vi "Read Motion Settings.vi"(8 "error in (no error)":errorcluster, 11 "Focus Class in":refnum<class "Focus Class.lvclass">) -> (0 "error out":errorcluster, 2 "Motion Settings":T1, 3 "Focus Class out":refnum<class "Focus Class.lvclass">)   [LabVIEW 2021, in "Focus Class.lvclass"]
uses:
  Focus Class.lvclass
  Focus cluster Motion Settings.ctl
  Focus Class.lvclass/Focus Class.ctl
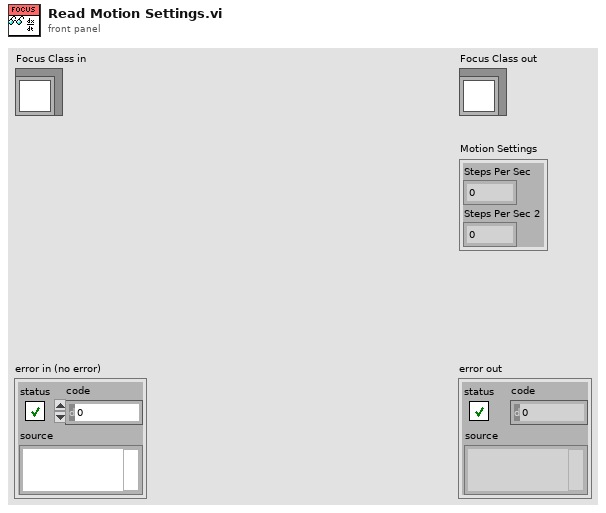
[diagram p1: front panel]
types:
  T1 = typedef "Focus cluster Motion Settings.ctl" = cluster{"Steps Per Sec":i32, "Steps Per Sec 2":i32}
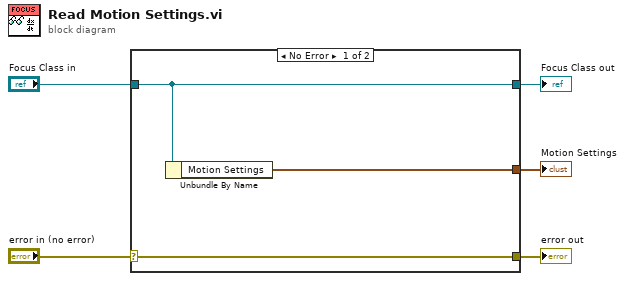
[diagram p0: block diagram]
diagram:
  n1 = case shown="No Error" "error in (no error)" {
    selector: "error in (no error)" -> [w8 w9]
    tunnel: [w8 w9] -> w4
    tunnel: [w7 w10] -> w2
    tunnel: "Focus Class in" -> [w7 w10]
    tunnel: [w6 _] -> w1
    frame No Error {
      n2 = Unbundle By Name(w7) -> ("Motion Settings"=w6:T1)
    }
    frame Error {
    }
  }
  "error out" <- w4
  "Focus Class out" <- w2
  "Motion Settings" <- w1
